vi "Check Plugin Active.vi"(8 "error in (no error)":errorcluster, 10 "Plugin":string, 11 "Execution UI in":refnum<class "Execution UI.lvclass">) -> (0 "error out":errorcluster, 2 "Active?":bool, 3 "Execution UI out":refnum<class "Execution UI.lvclass">)   [LabVIEW 2020, in "Execution UI.lvclass"]
uses:
  Execution UI.lvclass
  Execution UI.lvclass/Execution UI.ctl
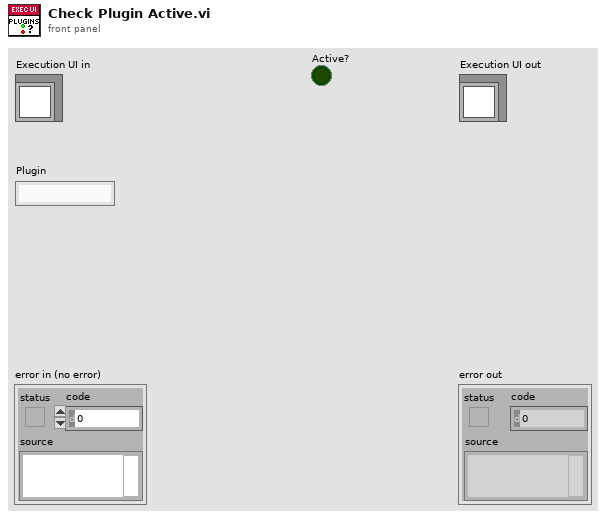
[diagram p1: front panel]
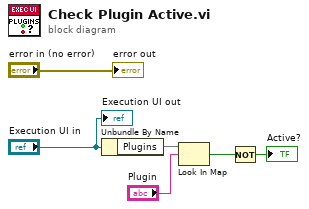
[diagram p0: block diagram]
diagram:
  n1 = Unbundle By Name("Execution UI in") -> ("Plugins"=w4:map{string, refnum<class "Plugin.lvclass">})
  n2 = Look In Map(map=w4, key="Plugin") -> (key not found?=w2:bool)  [unwired: 1 in, 1 out]
  n3 = Not(x=w2) -> (.not. x?=→"Active?":bool)
  "error out" <- "error in (no error)"
  "Execution UI out" <- "Execution UI in"
